vi "saveTargetsFile.vi"(5 "BL Targets":T1[](array[typedef])=[{"Code"="B2", "n"=0.23999999999999996, "Z:FS:(m)"=[15.0, 25.5], "U:FS:(m/s)"=[15.0, 25.5], "TI::(%)"=[15.0, 25.5]}, {"Code"="C2", "n"=0.14, "Z:FS:(m)"=[15.0, 16.0], "U:FS:(m/s)"=[15.0, 25.5], "TI::(%)"=[15.0, 25.5]}] {"n" min=0.02 max=0.5 step=0.01 format="%.2f"}, 7 "Path":path, 9 "ZrefMSmm":dbl, 10 "Scale":dbl=300.0 caption="Scale 1:" min=1.0 max=10000.0 step=50.0) -> ()   [LabVIEW 2021]
uses:
  BLTarget.ctl
panel:
  out "String":string
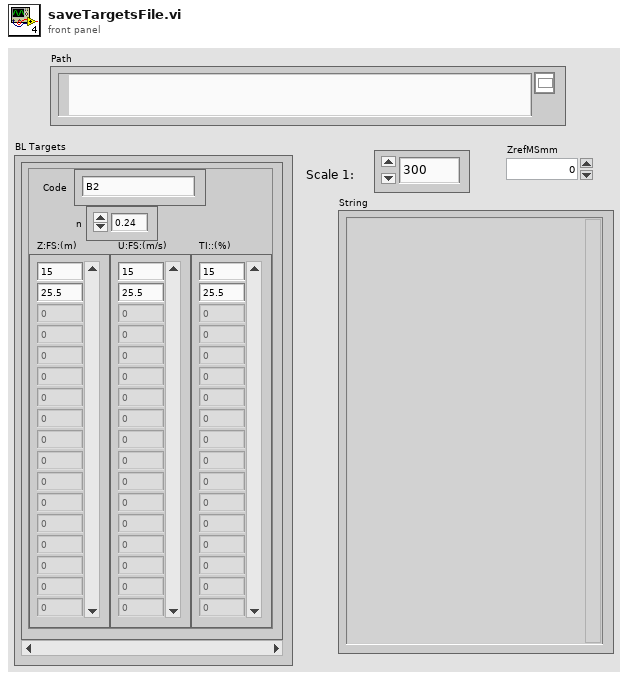
[diagram p1: front panel]
types:
  T1 = typedef "BLTarget.ctl" = cluster{"Code":string, "n":dbl, "Z:FS:(m)":dbl[], "U:FS:(m/s)":dbl[], "TI::(%)":dbl[]}
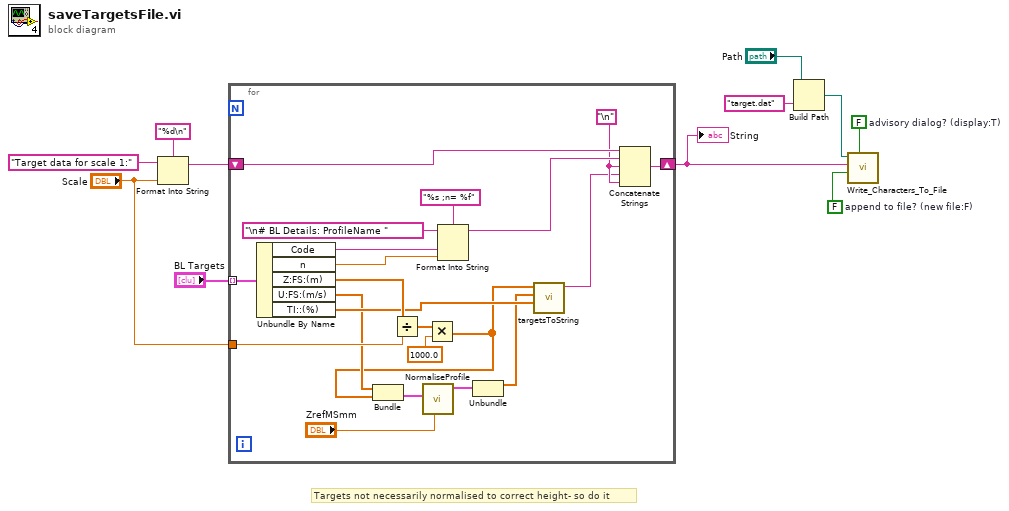
[diagram p0: block diagram]
diagram:
  w6 = FALSE  # advisory dialog? (display:T)
  w5 = FALSE  # append to file? (new file:F)
  # "Targets not necessarily normalised to correct height- so do it"
  n1 = Format Into String(format string="%d\n", initial string="Target data for scale 1:", "Scale") -> (resulting string=w8:string)  [unwired: 1 in, 1 out]
  n2 = for {
    tunnel: "BL Targets" -> [w32] mode=indexing
    shift-right: [w25] -> w2
    shift-left: w8 -> [w26]
    tunnel: "Scale" -> [w22]
    w21 = "\n"
    n3 = Unbundle By Name(w32) -> ("Code"=w31:string, "n"=w30:dbl, "Z:FS:(m)"=w20:dbl[], "U:FS:(m/s)"=w16:dbl[], "TI::(%)"=w19:dbl[])
    n4 = Divide(x=w20, y=w22) -> (x/y=w24:dbl[])
    n5 = Multiply(x=w24, y=1000.0) -> (x*y=w15:dbl[])
    n6 = Bundle("U:FS:(m/s)"=w16, w15) -> (w17:cluster{"U:FS:(m/s)":dbl[], dbl[]})  [unwired: 1 in]
    n7 = call "NormaliseProfile.vi"("Zref"="ZrefMSmm", "UzClusterIn"=w17) -> ("UzClusterOutput"=w13:cluster{dbl[], dbl[]})  [unwired: 8 in, 1 out]
    n8 = Format Into String(format string="%s ;n= %f", initial string="\n# BL Details: ProfileName ", w31, w30) -> (resulting string=w27:string)  [unwired: 1 in, 1 out]
    n9 = Unbundle(w13) -> (w12:dbl[])  [unwired: 1 out]
    n10 = call "targetsToString.vi"("Column3"=w19, "Column2"=w12, "Column1"=w15) -> ("plotString"=w18:string)  [unwired: 8 in]
    n11 = Concatenate Strings(w26, w27, w21, w18, w21) -> (w25:string)
  }
  "String" <- w2
  n12 = Build Path(base path="Path", name or relative path="target.dat") -> (appended path=w3:path)
  n13 = call "Write_Characters_To_File.vi"("file path (dialog if empty)"=w3, "advisory dialog? (display:T)"=w6, "character string"=w2, "append to file? (new file:F)"=w5) -> ()  [unwired: 1 in, 4 out]
